vi "MultiplexModbusRxData.vi"(10 "ID":u16, 11 "InputFIFO":refnum<k21>="ModbusSubnetERxDataFIFO") -> ()   [LabVIEW 2016]
uses:
  <vilib>/rvi/DataTransferAndStorage/Container/Common/niFpgaContainerExecOnDevCompGetState.vi
  <vilib>/rvi/Emulation/niFpgaEmulationIsFPGAContextNoSignature.vi
  <vilib>/rvi/Emulation/niFpgaSctlEmulationGetInTimedLoop.vi
  <vilib>/rvi/errors/niFpgaSetErrorForExecOnDevCompSimple.vi
  <vilib>/rvi/eio/common/nirviEmuReportErrorAndStop.vi
  <vilib>/rvi/DataTransferAndStorage/Container/Common/niFpgaContainerGetUniqueNameForEmu.vi
  <vilib>/rvi/FIFO/Fifo_Resource/nirvififoEmulationSetSize.vi
  <vilib>/rvi/FIFO/Fifo_Resource/nirviFifoEmulationQueueMgr.vi
  <instcachedir>/0/nirviFifoEmulationQueueMgr_E5CAEC123FF24DC58D834DCA3CDAA9B5.lvgen/nirviFifoEmulationQueueMgr_E5CAEC123FF24DC58D834DCA3CDAA9B5_002.vi
  <vilib>/rvi/FIFO/Fifo_Resource/nirvififoEmulationDetermineInputValidOut.vi
  <vilib>/rvi/FIFO/Fifo_Resource/nirvififoEmulationCreateLock.vi
  <vilib>/rvi/Emulation/niFpgaProcessEmulError.vi
  <vilib>/rvi/FIFO/Fifo_Resource/nirvififoEmulationObtainLock.vi
  <vilib>/rvi/FIFO/Fifo_Resource/nirvififoEmulationReleaseLock.vi
  <vilib>/rvi/occurrence/nirviWaitOnOccurrenceBase.vi
  <vilib>/rvi/errors/nirviReportUnexpectedCaseInternalError.vi
  <vilib>/rvi/errors/nirviReportUnexpectedCaseInternalError (U32).vi
  <vilib>/Utility/error.llb/Clear Errors.vi
  <vilib>/rvi/interface/RandomDataEmulation/niFpgaRandomDataHandleErrors.vi
  <vilib>/rvi/Emulation/niFpgaGetClockAttributes.vi
  <vilib>/rvi/Emulation/niFpgaEmulationReportErrorSimple.vi
  <vilib>/rvi/Emulation/niFpgaCriticalErrorInLSC.vi
  <vilib>/rvi/DataTransferAndStorage/Container/XNode/niFpgaContainer.xnode
  <vilib>/rvi/FIFO/Fifo_Resource/niFpgaFifoEmulationRefIn.vi
  <vilib>/rvi/FIFO/Fifo_Resource/nirvififoEmulationWrite.vi
  <vilib>/rvi/interface/RandomDataEmulation/nirviRandomDataFpgaReadWriteTemplate.vi
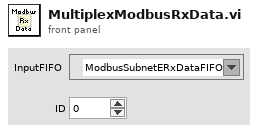
[diagram p1: front panel]
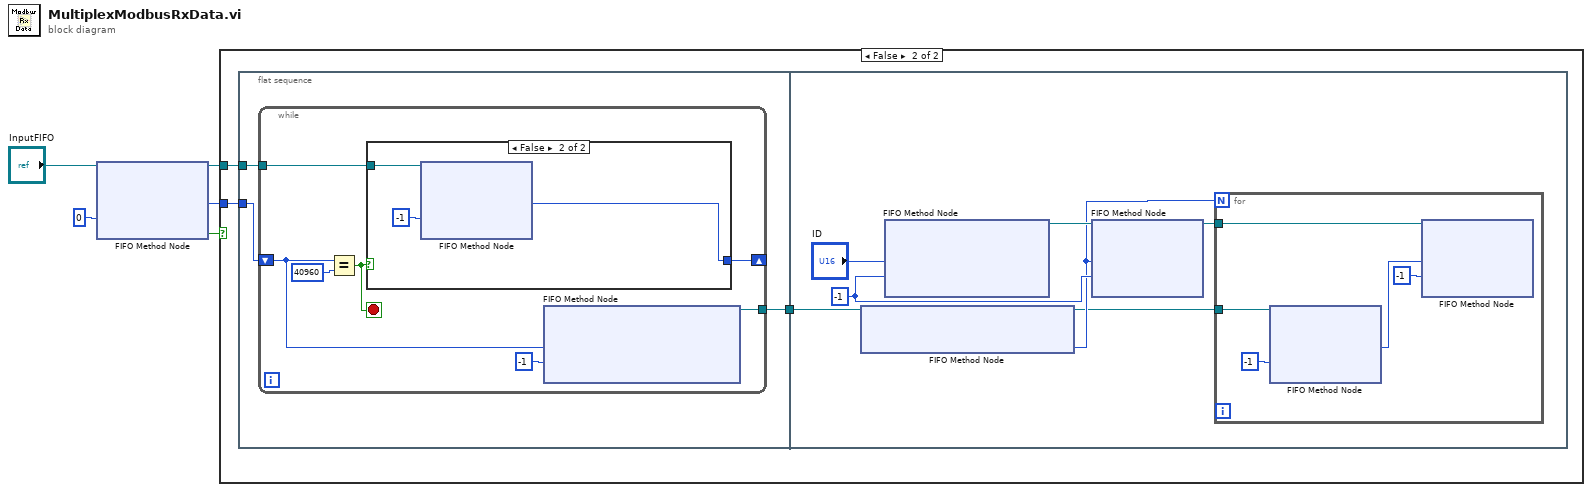
[diagram p0: block diagram]
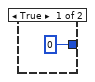
[diagram p3: hidden frame]
diagram:
  n1 = xnode ("FIFO Method Node")("Timeout"=0, "FIFO In"="InputFIFO") -> ("Element"=w4:u16, "Timed Out?"=w5:bool, "FIFO Out"=w2:refnum<k21>)
  n2 = case shown="False" w5 {
    tunnel: w4 -> [_ w7]
    tunnel: w2 -> [_ w8]
    frame True {
    }
    frame False {
      n3 = flat-sequence {
        tunnel: w8 -> [w11]
        tunnel: w7 -> [w10]
        tunnel: [w9] -> w6
        tunnel: w6 -> [w25]
        frame #0 {
          n4 = while {
            shift-right: [w17] -> _
            shift-left: w10 -> [w16]
            tunnel: w11 -> [w12]
            tunnel: [w13] -> w9
            stop <- w14 stop-if-true
            n5 = Equal?(x=w16, y=u16 40960) -> (x = y?=w14:bool)
            n6 = case shown="False" w14 {
              tunnel: [u16 0 ("Element") w22] -> w17
              tunnel: w12 -> [_ w20]
              frame True {
              }
              frame False {
                n7 = xnode ("FIFO Method Node")("Timeout"=-1, "FIFO In"=w20) -> ("Element"=w22:u16)  [unwired: 2 out]
              }
            }
            n8 = xnode ("FIFO Method Node")("Element"=w16, "Timeout"=-1) -> ("FIFO Out"=w13:refnum<k21>)  [unwired: 1 in, 1 out]
          }
        }
        frame #1 {
          w28 = -1 ("Timeout")
          n9 = xnode ("FIFO Method Node")("FIFO In"=w25) -> ("Number of Elements to Read"=w26:u32, "FIFO Out"=w24:refnum<k21>)
          n10 = xnode ("FIFO Method Node")("Element"="ID", "Timeout"=w28) -> ("FIFO Out"=w27:refnum<k21>)  [unwired: 1 in, 1 out]
          n11 = xnode ("FIFO Method Node")("Element"=w26, "Timeout"=w28, "FIFO In"=w27) -> ("FIFO Out"=w23:refnum<k21>)  [unwired: 1 out]
          n12 = for {
            N: w26 -> [_]
            tunnel: w24 -> [w31]
            tunnel: w23 -> [w30]
            n13 = xnode ("FIFO Method Node")("Timeout"=-1, "FIFO In"=w31) -> ("Element"=w34:u16)  [unwired: 2 out]
            n14 = xnode ("FIFO Method Node")("Element"=w34, "Timeout"=-1, "FIFO In"=w30) -> ()  [unwired: 2 out]
          }
        }
      }
    }
  }
